vi "Current to totes VI.vi"() -> (3 "NumTotes":dbl)   [LabVIEW 2014]
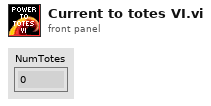
[diagram p1: front panel]
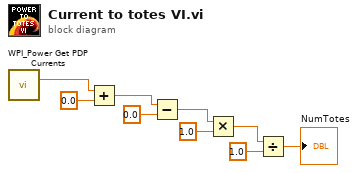
[diagram p0: block diagram]
diagram:
  n1 = call <vilib>:"WPI_Power Get PDP Currents.vi"() -> ("current (A)"=w6:dbl)  [unwired: 13 in, 2 out]
  n2 = Add(x=w6, y=0.0) -> (x+y=w7:dbl)
  n3 = Subtract(x=w7, y=0.0) -> (x-y=w8:dbl)
  n4 = Multiply(x=w8, y=1.0) -> (x*y=w9:dbl)
  n5 = Divide(x=w9, y=1.0) -> (x/y=→"NumTotes":dbl)
